vi "Save Setting to DB.vi"(8 "error in (no error)":errorcluster, 10 "Array":string[](array[string]), 11 "Cluster":T1) -> (0 "error out":errorcluster)   [LabVIEW 2017]
uses:
  Controls/Testscreen_Input cluster.ctl
  <vilib>/addons/database/Connection.llb/Conn ObjectReference.ctl
  <vilib>/addons/database/NI_Database_API.lvlib
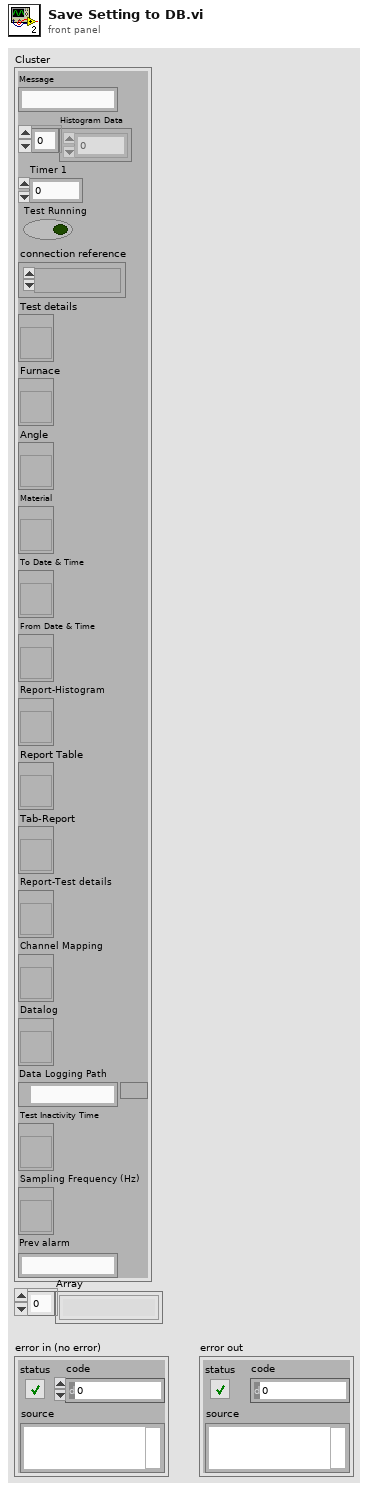
[diagram p1: front panel]
types:
  T1 = typedef "Testscreen_Input cluster.ctl" = cluster{"Message":string, "Histogram Data":i32[], "Timer 1":u32, "Test Running":bool, "connection reference":T2, "Test details":refnum<vi>, "Furnace":refnum<vi>, "Angle":refnum<vi>, "Material":refnum<vi>, "To Date & Time":refnum<vi>, "From Date & Time":refnum<vi>, "Report-Histogram":refnum<vi>, "Report Table":refnum<vi>, "Tab-Report":refnum<vi>, "Report-Test details":refnum<vi>, "Channel Mapping":refnum<vi>, "Datalog":refnum<vi>, "Data Logging Path":path, "Test Inactivity Time":refnum<vi>, "Sampling Frequency (Hz)":refnum<vi>, "Prev alarm":string}
  T2 = typedef "NI_Database_API.lvlib/Conn ObjectReference.ctl" = refnum<k1>
  T3 = cluster{"String":string, "Sampling Frequency (Hz)":string}
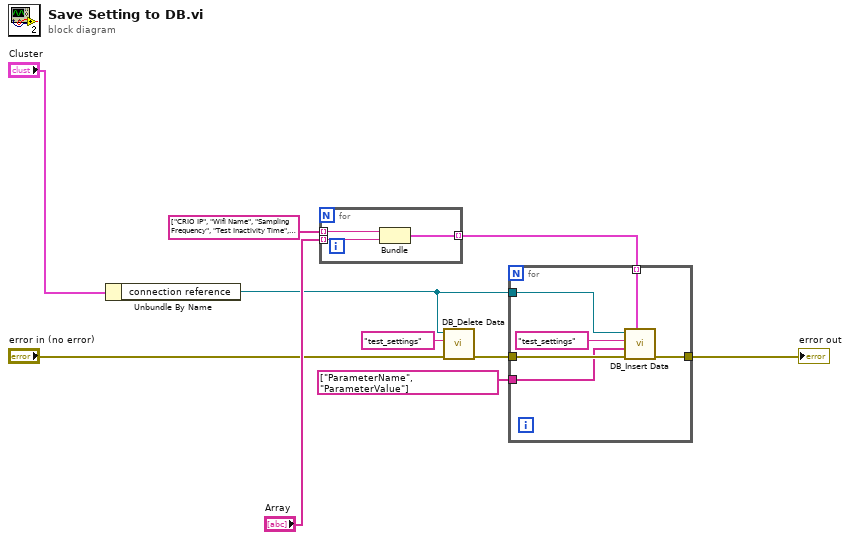
[diagram p0: block diagram]
diagram:
  n1 = Unbundle By Name("Cluster") -> ("connection reference"=w2:T2)
  n2 = for {
    tunnel: string[] ["CRIO IP", "Wifi Name", "Sampling Frequency", "Test Inactivity Time", "Drive Path"] ("columns") -> [w13] mode=indexing
    tunnel: "Array" -> [w12] mode=indexing
    tunnel: [w11] -> w8 mode=indexing
    n3 = Bundle("String"=w13, "Sampling Frequency (Hz)"=w12) -> (w11:T3)  [unwired: 1 in]
  }
  n4 = call "DB_Delete Data.vi"("error in (no error)"="error in (no error)", "table"="test_settings", "connection reference"=w2) -> ("error out"=w3:errorcluster)  [unwired: 8 in]
  n5 = for {
    tunnel: w2 -> [w17]
    tunnel: string[] ["ParameterName", "ParameterValue"] ("table") -> [w15]
    tunnel: w3 -> [w16]
    tunnel: [w19] -> w10
    tunnel: w8 -> [w14] mode=indexing
    n6 = call "DB_Insert Data.vi"("data"=w14, "error in (no error)"=w16, "columns"=w15, "table"="test_settings", "connection reference"=w17) -> ("error out"=w19:errorcluster)  [unwired: 6 in]
  }
  "error out" <- w10
